vi "get images.vi"(8 "error in (no error)":errorcluster, 11 "Room in":refnum<class "Room.lvclass">) -> (0 "error out":errorcluster, 2 "images":T1[](array[typedef]), 3 "Room out":refnum<class "Room.lvclass">)   [LabVIEW 2016, in "Room.lvclass"]
uses:
  Room.lvclass
  <vilib>/picture/picture.llb/imagedata.ctl
  Room.lvclass/Room.ctl
  MapSite/MapSite.lvclass
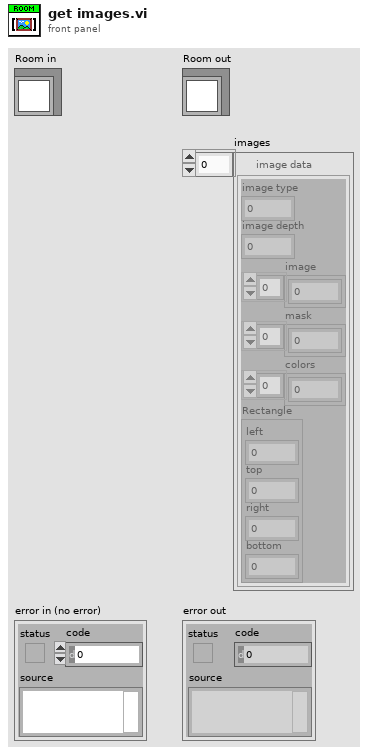
[diagram p1: front panel]
types:
  T1 = typedef "imagedata.ctl" = cluster{"image type":i32, "image depth":i32, "image":u8[], "mask":u8[], "colors":u32[], "Rectangle":cluster{"left":i16, "top":i16, "right":i16, "bottom":i16}}
  T2 = cluster{"left":i16, "top":i16, "right":i16, "bottom":i16}
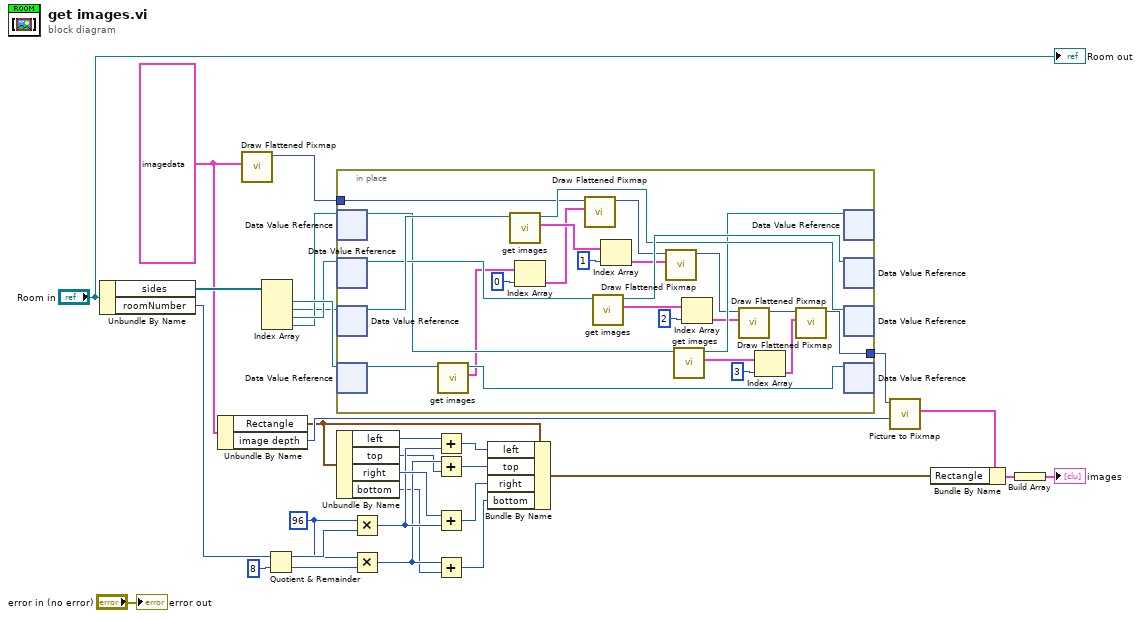
[diagram p0: block diagram]
diagram:
  w1 = 96 ("y")
  w22 = T1 {"image type"=0, "image depth"=24, "image"=array[27648 elements], "mask"=[], "colors"=[], "Rectangle"={"left"=0, "top"=0, "right"=96, "bottom"=96}} ("image data")
  n1 = Unbundle By Name("Room in") -> ("sides"=w29:refnum<data-value>[], "roomNumber"=w19:i32)
  n2 = Unbundle By Name(w22) -> ("Rectangle"=w13:T2, "image depth"=w21:i32)
  n3 = call <vilib>:"Draw Flattened Pixmap.vi"("image data"=w22) -> ("new picture"=w24:picture)  [unwired: 8 in]
  n4 = Index Array(array=w29) -> (element #1=w28:refnum<data-value>, element #2=w25:refnum<data-value>, element #3=w27:refnum<data-value>, element #4=w26:refnum<data-value>)  [unwired: 4 in]
  n5 = Quotient & Remainder(x=w19, y=8) -> (x-y*floor(x/y)=w17:i32, floor(x/y)=w10:i32)
  n6 = in-place {
    in-place-border: w24 -> [w39]
    in-place-border: [w32] -> w23
    n7 = in-place-dvr #1(w26) -> (w50:refnum<class "MapSite.lvclass">)  [unwired: 1 out]
    n8 = in-place-dvr #2(w27) -> (w53:refnum<class "MapSite.lvclass">)  [unwired: 1 out]
    n9 = in-place-dvr #3(w25) -> (w55:refnum<class "MapSite.lvclass">)  [unwired: 1 out]
    n10 = in-place-dvr #4(w28) -> (w56:refnum<class "MapSite.lvclass">)  [unwired: 1 out]
    n11 = call-dynamic "get images.vi"("MapSite in"=w56) -> ("images"=w48:T1[], "MapSite out"=w54:refnum<class "MapSite.lvclass">)  [unwired: 8 in, 1 out]
    n12 = call-dynamic "get images.vi"("MapSite in"=w55) -> ("images"=w47:T1[], "MapSite out"=w51:refnum<class "MapSite.lvclass">)  [unwired: 8 in, 1 out]
    n13 = Index Array(array=w48, index=0) -> (element=w40:T1)
    n14 = call <vilib>:"Draw Flattened Pixmap.vi"("image data"=w40, "picture"=w39) -> ("new picture"=w38:picture)  [unwired: 7 in]
    n15 = call-dynamic "get images.vi"("MapSite in"=w53) -> ("images"=w46:T1[], "MapSite out"=w52:refnum<class "MapSite.lvclass">)  [unwired: 8 in, 1 out]
    n16 = Index Array(array=w47, index=1) -> (element=w35:T1)
    n17 = call <vilib>:"Draw Flattened Pixmap.vi"("image data"=w35, "picture"=w38) -> ("new picture"=w37:picture)  [unwired: 7 in]
    n18 = call-dynamic "get images.vi"("MapSite in"=w50) -> ("images"=w45:T1[], "MapSite out"=w49:refnum<class "MapSite.lvclass">)  [unwired: 8 in, 1 out]
    n19 = Index Array(array=w46, index=2) -> (element=w34:T1)
    n20 = call <vilib>:"Draw Flattened Pixmap.vi"("image data"=w34, "picture"=w37) -> ("new picture"=w36:picture)  [unwired: 7 in]
    n21 = Index Array(array=w45, index=3) -> (element=w33:T1)
    n22 = call <vilib>:"Draw Flattened Pixmap.vi"("image data"=w33, "picture"=w36) -> ("new picture"=w32:picture)  [unwired: 7 in]
    n23 = in-place-dvr #1(w49) -> ()  [unwired: 2 out]
    n24 = in-place-dvr #2(w52) -> ()  [unwired: 2 out]
    n25 = in-place-dvr #3(w51) -> ()  [unwired: 2 out]
    n26 = in-place-dvr #4(w54) -> ()  [unwired: 2 out]
  }
  n27 = Unbundle By Name(w13) -> ("left"=w16:i16, "top"=w8:i16, "right"=w15:i16, "bottom"=w7:i16)
  n28 = Multiply(x=w1, y=w17) -> (x*y=w14:i32)
  n29 = Multiply(x=w1, y=w10) -> (x*y=w9:i32)
  n30 = Add(x=w16, y=w14) -> (x+y=w12:i32)
  n31 = Add(x=w9, y=w8) -> (x+y=w6:i32)
  n32 = Add(x=w15, y=w14) -> (x+y=w11:i32)
  n33 = Add(x=w9, y=w7) -> (x+y=w5:i32)
  n34 = Bundle By Name(cluster=w13, "left"=w12, "top"=w6, "right"=w11, "bottom"=w5) -> (w3:T2)
  n35 = call <vilib>:"Picture to Pixmap.vi"("depth"=w21, "picture"=w23) -> ("image data"=w4:T1)  [unwired: 8 in, 1 out]
  n36 = Bundle By Name(cluster=w4, "Rectangle"=w3) -> (w2:T1)
  n37 = Build Array(w2) -> (→"images":T1[])
  "error out" <- "error in (no error)"
  "Room out" <- "Room in"
